vi "AKIP_reset_errors.vi"(8 "error in (no error)":errorcluster, 11 "VISA Refnum in":refnum<visa-resource-name>="AKIP") -> (0 "error out":errorcluster, 3 "VISA Refnum out":refnum<visa-resource-name>)   [LabVIEW 2017]
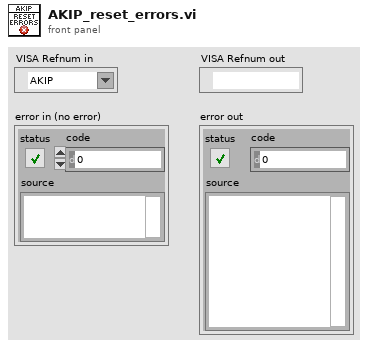
[diagram p1: front panel]
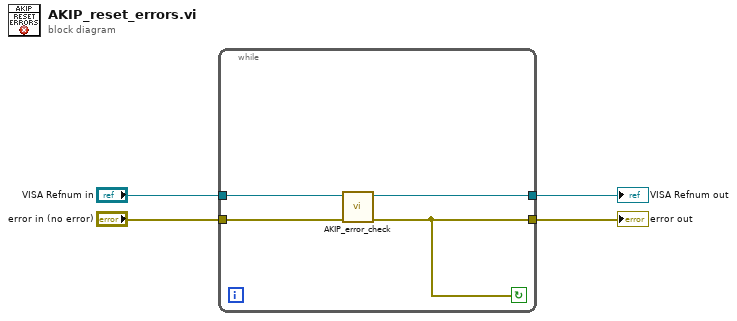
[diagram p0: block diagram]
diagram:
  n1 = while {
    tunnel: "VISA Refnum in" -> [w7]
    tunnel: "error in (no error)" -> [w8]
    tunnel: [w6] -> w2
    tunnel: [w5] -> w1
    stop <- w5 continue-if-true
    n2 = call "AKIP_error_check.vi"("error in (no error)"=w8, "VISA Refnum in"=w7) -> ("error out"=w5:errorcluster, "VISA Refnum out"=w6:refnum<visa-resource-name>)  [unwired: 8 in]
  }
  "error out" <- w1
  "VISA Refnum out" <- w2
